vi "Autotest_Instr.vi"(8 "error in (no error)":errorcluster caption="entrée d'erreur (pas d'erreur)", 11 "Class Relay_Board en entrée":refnum<class "Class Instrument Relay_Board.lvclass">) -> (0 "error out":errorcluster caption="sortie d'erreur", 3 "Class Relay_Board en Sortie":refnum<class "Class Instrument Relay_Board.lvclass">)   [LabVIEW 2020, in "Library Instrument & Equipement.lvlib" / "Library Instruments.lvlib" / "Class Instrument Relay_Board.lvclass"]
uses:
  Class Instrument Relay_Board.lvclass
  C:/Users/ngarcin/OneDrive - Altyor/Standard TB/Class/Instrument/Instrument (Default)/Class Instrument (Default).lvclass
  Class Instrument Relay_Board.lvclass/Class Instrument Relay_Board.ctl
  Instrument (Default)/Class Instrument (Default).lvclass
  Relay_Board/Relay_Board (Default)/Class Relay_Board (Default).lvclass
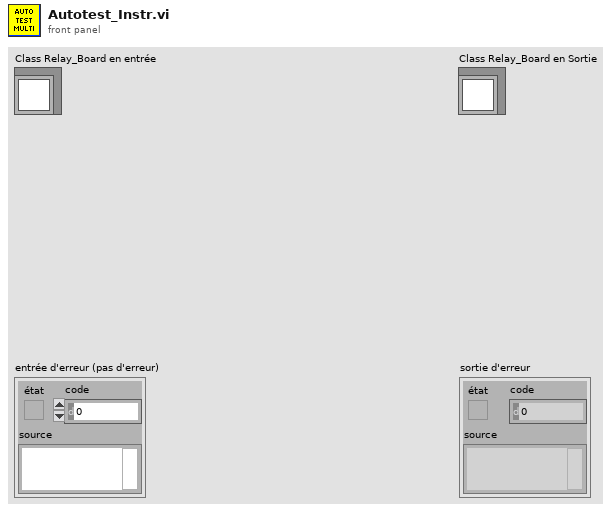
[diagram p1: front panel]
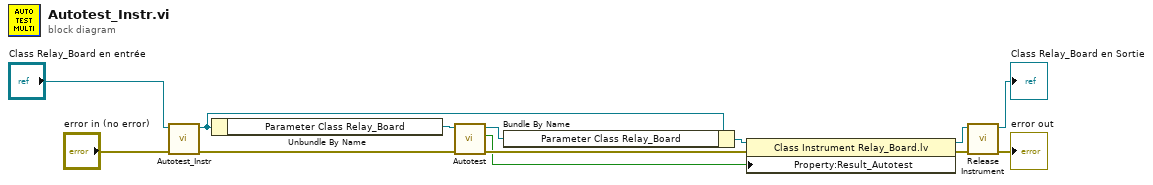
[diagram p0: block diagram]
diagram:
  n1 = call-parent "Autotest_Instr.vi"("error in (no error)"="error in (no error)", "Class Instrument (Default) en entrée"="Class Relay_Board en entrée") -> ("error out"=w10:errorcluster, "Class Instrument (Default) en sortie"=w11:refnum<class "Class Instrument Relay_Board.lvclass">)  [unwired: 8 in]
  n2 = Unbundle By Name(w11) -> ("Parameter Class Relay_Board"=w9:refnum<class "Class Relay_Board (Default).lvclass">)
  n3 = call-dynamic "Autotest.vi"("error in (no error)"=w10, "Class Relay_Board (Default) en entrée"=w9) -> ("error out"=w7:errorcluster, "Autotest Ok ?"=w5:bool, "Class Relay_Board (Default) en sortie"=w8:refnum<class "Class Relay_Board (Default).lvclass">)  [unwired: 7 in]
  n4 = Bundle By Name(cluster=w11, "Parameter Class Relay_Board"=w8) -> (w6:refnum<class "Class Instrument Relay_Board.lvclass">)
  n5 = property class="Class Instrument Relay_Board.lv"(reference=w6, error in=w7, "Property:Result_Autotest"=w5) -> (reference out=w2:refnum<class "Class Instrument Relay_Board.lvclass">, error out=w4:errorcluster)
  n6 = call-dynamic "Release Instrument.vi"("error in (no error)"=w4, "Class Instrument (Default) en entrée"=w2) -> ("error out"=→"error out":errorcluster, "Class Instrument (Default) en sortie"=→"Class Relay_Board en Sortie":refnum<class "Class Instrument Relay_Board.lvclass">)  [unwired: 8 in]
